vi "Close Azure Session.vi"(8 "error in (no error)":errorcluster, 11 "Azure Session":refnum<class "Session.lvclass">) -> (0 "error out":errorcluster)   [LabVIEW 2015, in "NI_Azure_Core.lvlib" / "Session.lvclass"]
doc: "Close the specified Azure session."
uses:
  Session.lvclass
  Session.lvclass/Session.ctl
  Read HTTP Session.vi
  <vilib>/httpClient/LabVIEWHTTPClient.lvlib
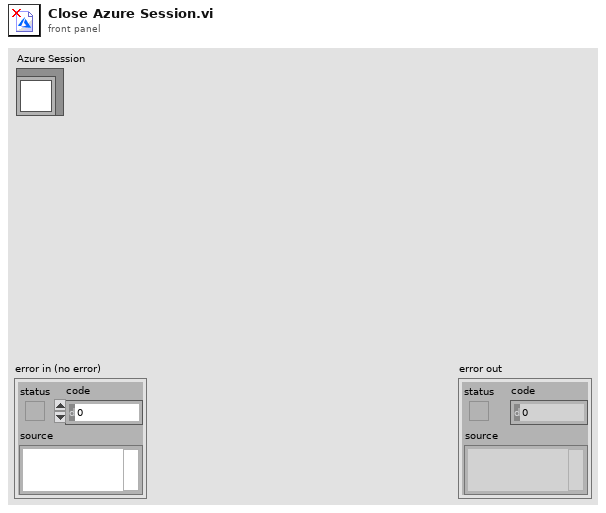
[diagram p1: front panel]
types:
  T1 = typedef "LabVIEWHTTPClient.lvlib/ClientHandle.ctl" = refnum<k1>
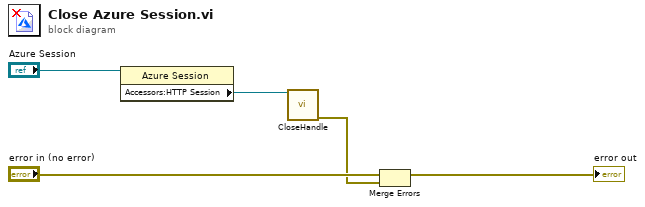
[diagram p0: block diagram]
diagram:
  n1 = property class="Azure Session"(reference="Azure Session") -> ("Accessors:HTTP Session"=w3:T1)  [unwired: 1 in, 2 out]
  n2 = call <vilib>:"CloseHandle.vi"("client handle"=w3) -> ("error out"=w1:errorcluster)  [unwired: 14 in]
  n3 = Merge Errors("error in (no error)", w1) -> (→"error out":errorcluster)
